vi "setUp.vi"(8 "error in (no error)":errorcluster) -> (0 "error out":errorcluster, 2 "connection ID":refnum<k5>, 3 "session":T1)   [LabVIEW 2013, in "support.lvlib"]
doc: "Initialize the library, open a connection and authenticate a session with the SSH server."
uses:
  libssh2/Session Refnum.ctl
  libssh2/libssh2_init_default.vi
  libssh2/libssh2_session_handshake_tcp.vi
  support.lvlib
  libssh2/libssh2.lvlib
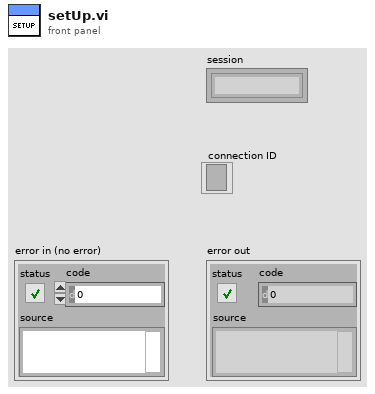
[diagram p1: front panel]
types:
  T1 = typedef "libssh2.lvlib/Session Refnum.ctl" = refnum<k1>
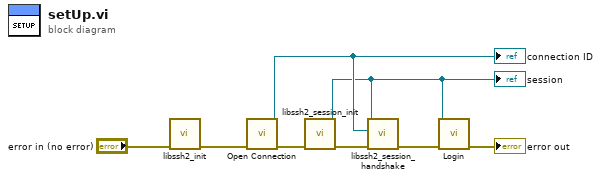
[diagram p0: block diagram]
diagram:
  n1 = call-poly "libssh2_init.vi"("error in (no error)"="error in (no error)") -> ("error out"=w7:errorcluster)  [unwired: 10 in]
  n2 = call "Open Connection.vi"("error in (no error)"=w7) -> ("error out"=w8:errorcluster, "connection ID"=w6:refnum<k5>)  [unwired: 9 in]
  "connection ID" <- w6
  n3 = call "libssh2_session_init.vi"("error in (no error)"=w8) -> ("error out"=w3:errorcluster, "session"=w4:T1)  [unwired: 9 in]
  "session" <- w4
  n4 = call-poly "libssh2_session_handshake.vi"("error in (no error)"=w3, "tcp connection"=w6, "session"=w4) -> ("error out"=w5:errorcluster)  [unwired: 8 in]
  n5 = call "Login.vi"("error in (no error)"=w5, "session"=w4) -> ("error out"=→"error out":errorcluster)  [unwired: 9 in]
